vi "InitAppearance.vi"(7 "Col Array Ref in":refnum<vi>, 8 "error in (no error)":errorcluster, 9 "Table Ref in":refnum<vi>, 10 "Col #":i32, 11 "MenuDisableCol in":refnum<class "MenuDisableCol.lvclass">) -> (0 "error out":errorcluster, 1 "Table Ref out":refnum<vi>, 3 "MenuDisableCol out":refnum<class "MenuDisableCol.lvclass">, 4 "Needs 2nd pass":bool)   [LabVIEW 2013, in "MenuDisableCol.lvclass"]
doc: "Set column header, width, background and text color for entire table column."
uses:
  MenuDisableCol.lvclass
  <vilib>/Utility/miscctls.llb/LVRowAndColumnTypeDef.ctl
  MenuCol/MenuCol.lvclass
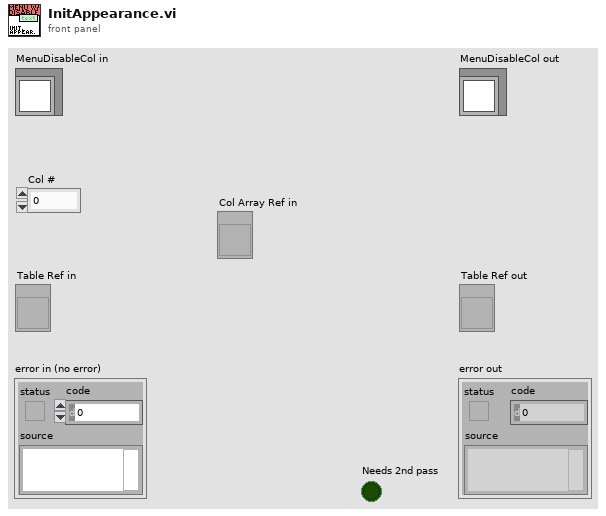
[diagram p1: front panel]
types:
  T1 = typedef "LVRowAndColumnTypeDef.ctl" = cluster{"Row":i32, "Column":i32}
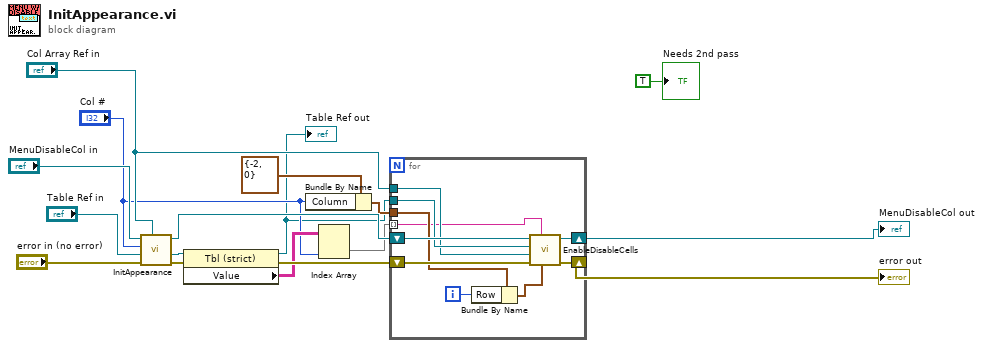
[diagram p0: block diagram]
diagram:
  n1 = call-parent "InitAppearance.vi"("Col Array Ref in"="Col Array Ref in", "error in (no error)"="error in (no error)", "Table Ref in"="Table Ref in", "Col #"="Col #", "Column in"="MenuDisableCol in") -> ("error out"=w12:errorcluster, "Table Ref out"=w13:refnum<vi>, "Column out"=w10:refnum<class "MenuDisableCol.lvclass">)  [unwired: 3 in, 1 out]
  n2 = property class="Tbl (strict)"(reference=w13, error in=w12) -> (reference out=w2:refnum<vi>, error out=w9:errorcluster, "Value"=w6:string[][])
  "Table Ref out" <- w2
  n3 = Bundle By Name(cluster=T1 {"Row"=-2, "Column"=0} ("RowAndCollumn"), "Column"="Col #") -> (w7:T1)
  n4 = Index Array(array=w6, index (col)="Col #") -> (element=w4:string[])  [unwired: 1 in]
  n5 = for {
    tunnel: w2 -> [w26]
    tunnel: "Col Array Ref in" -> [w24]
    tunnel: w7 -> [w23]
    shift-right: [w21] -> w1
    shift-left: w9 -> [w25]
    tunnel: w4 -> [w19] mode=indexing
    shift-right: [w18] -> w3
    shift-left: w10 -> [w27]
    i -> [w20]
    n6 = Bundle By Name(cluster=w23, "Row"=w20) -> (w22:T1)
    n7 = call-dynamic "EnableDisableCells.vi"("Cell Position"=w22, "Item Name or Tag"=w19, "error in (no error)"=w25, "Col Array Ref in"=w24, "Table CtlRef in"=w26, "MenuDisableCol in"=w27) -> ("error out"=w21:errorcluster, "MenuDisableCol out"=w18:refnum<class "MenuDisableCol.lvclass">)  [unwired: 2 in, 2 out]
  }
  "error out" <- w1
  "MenuDisableCol out" <- w3
  "Needs 2nd pass" <- TRUE ("Needs 2nd pass")
